vi "Check Aircraft Heartbeat.vi"(8 "error in (no error)":errorcluster, 11 "Aircraft ID":u8) -> (0 "Error Out":errorcluster)   [LabVIEW 2014]
uses:
  Aircraft Information/Sub VI/Get Aircraft Information.vi
  Aircraft Information/Sub VI/Set Aircraft Information.vi
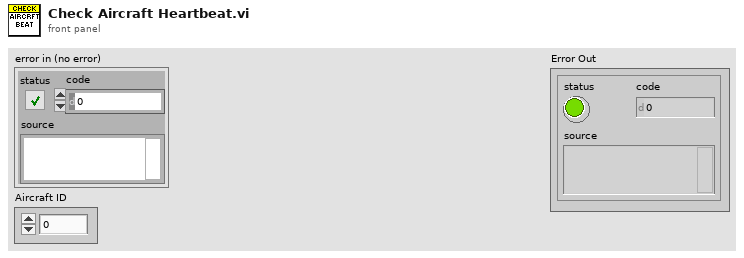
[diagram p1: front panel]
types:
  T1 = typedef "Drone Information.ctl" = cluster{"Aircraft ID":u8, "Tag ID":string, "System Status":string, "Base Mode":T2, "Armed/Disarmed":bool, "Battery Voltage":dbl, "Control Mode":T3, "Initialisation":u8, "Coms with aircraft good":bool, "Mode":string, "Mission Uploaded":bool}
  T2 = typedef "Base Mode.ctl" = cluster{"Custom Mode":bool, "Test Enabled":bool, "Autonomous Mode":bool, "Guided Mode":bool, "Stabilization Enabled":bool, "HIL Enabled":bool, "Manual Mode":bool, "Arm":bool}
  T3 = typedef "Aircraft Mode.ctl" = enum16{"Loiter", "Stabalise", "Failsafe", "Emergency Stop"}
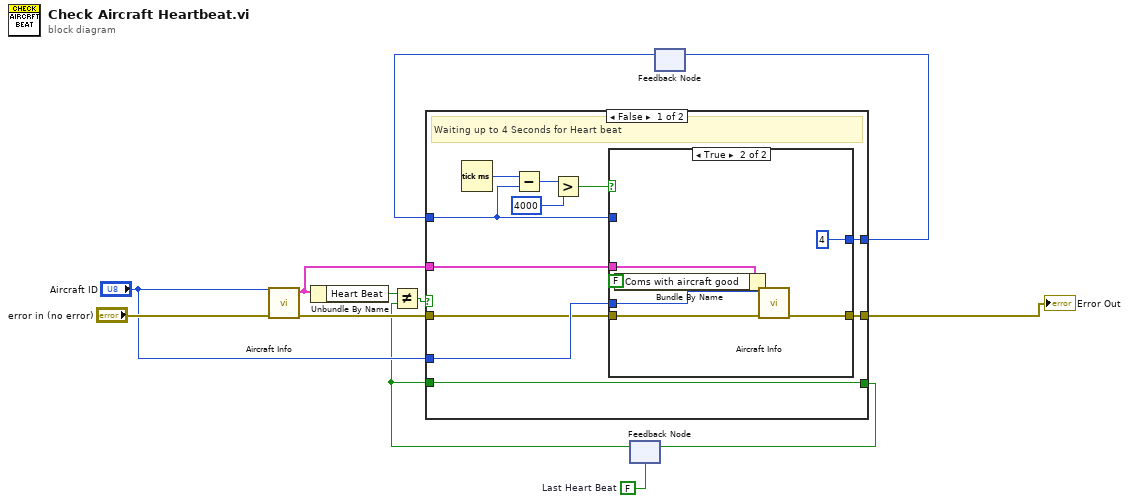
[diagram p0: block diagram]
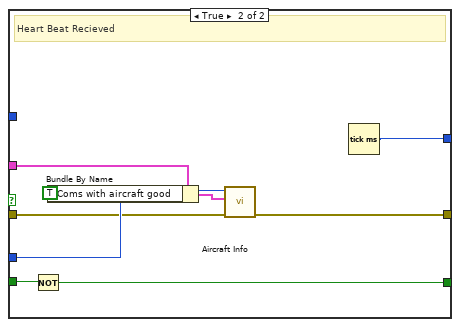
[diagram p3: hidden frame]
diagram:
  w3 = FALSE  # Last Heart Beat
  n1 = call-poly "Aircraft Info.vi"("Error In"="error in (no error)", "Aircraft ID"="Aircraft ID") -> ("Error Out"=w6:errorcluster, "Aircraft Information Out"=w9:T1)  [unwired: 8 in]
  n2 = Unbundle By Name(w9) -> ("Heart Beat"=w7:bool)
  n3 = feedback #1(w3) -> (w1:bool)
  n4 = Not Equal?(x=w7, y=w1) -> (x != y?=w8:bool)
  n5 = feedback #2() -> (w4:u32)  [unwired: 1 in]
  n6 = case shown="False" w8 {
    tunnel: w9 -> [w21 w38]
    tunnel: w1 -> [w23 w41]
    tunnel: [w23 w40] -> w2
    tunnel: w4 -> [w13 _]
    tunnel: [w20 w33] -> w5
    tunnel: w6 -> [w19 w35]
    tunnel: "Aircraft ID" -> [w22 w39]
    tunnel: [w18 w34] -> w10
    frame False {
      # "Waiting up to 4 Seconds for Heart beat"
      n7 = Tick Count (ms)() -> (millisecond timer value=w17:u32)
      n8 = Subtract(x=w17, y=w13) -> (x-y=w16:u32)
      n9 = Greater?(x=w16, y=u32 4000) -> (0:w14:bool)
      n10 = case shown="True" w14 {
        tunnel: w22 -> [_ w32]
        tunnel: w21 -> [_ w31]
        tunnel: [w25 4] -> w20
        tunnel: w13 -> [w25 _]
        tunnel: w19 -> [w24 w27]
        tunnel: [w24 w26] -> w18
        frame False {
        }
        frame True {
          n11 = Bundle By Name(cluster=w31, "Coms with aircraft good"=FALSE ("Heart Beat Status")) -> (w28:T1)
          n12 = call-poly "Aircraft Info.vi"("Error In"=w27, 10:w28, "Aircraft Information In"=w32) -> ("Error Out"=w26:errorcluster)  [unwired: 7 in, 1 out]
        }
      }
    }
    frame True {
      # "Heart Beat Recieved"
      n13 = Not(x=w41) -> (.not. x?=w40:bool)
      n14 = Bundle By Name(cluster=w38, "Coms with aircraft good"=TRUE ("Heart Beat Status")) -> (w36:T1)
      n15 = call-poly "Aircraft Info.vi"("Error In"=w35, 10:w36, "Aircraft Information In"=w39) -> ("Error Out"=w34:errorcluster)  [unwired: 7 in, 1 out]
      n16 = Tick Count (ms)() -> (millisecond timer value=w33:u32)
    }
  }
  "Error Out" <- w10
  n17 = feedback-in #1(w2) -> ()
  n18 = feedback-in #2(w5) -> ()
